vi "Measure Resistance (2 or 4-wire)_demo.vi"() -> ()   [LabVIEW 2013]
doc: "This example acquires a single Resistance measurement. Set the measurement type to either a 2-wire or 4-wire resistance measurement. Specify the range and absolute resolution of your input signal. The measured value will be displayed in the Measurement indicator. A Boolean indicator will indicate if the measured value is out of range."
uses:
  <instrlib>/niDMM/nidmm.llb/niDMM Function.ctl
  <instrlib>/niDMM/nidmm.llb/niDMM Resolution in Digits.ctl
  <instrlib>/niDMM/nidmm.llb/niDMM Offset Comp Ohms.ctl
  <instrlib>/niDMM/nidmm.llb/niDMM Configure Measurement Digits.vi
panel:
  out "Configuration:Range":dbl
  in  "Resolution in Digits":T1=5.5 items=["3 1/2"=3.5, "4 1/2"=4.5, "5 1/2"=5.5, "6 1/2"=6.5, "7 1/2"=7.5]
  out "Signal Out of Range":bool
  in  "Measurement Type":T2=enum."4-wire Resistance"
  in  "Device Name":refnum<k15>="4082_0"
  in  "Range (Ohms)":dbl=100.0 format="%.2p"
  out "Measurement (Ohms)":dbl format="%_7p"
  # "For instructions select File >> VI Properties >> Documentation"
  # "Configuration"
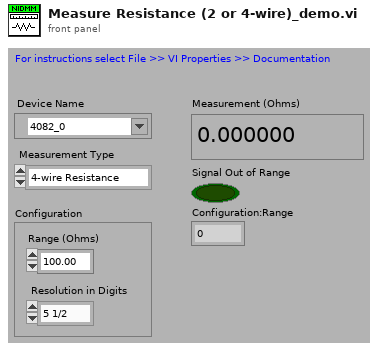
[diagram p1: front panel]
types:
  T1 = typedef "niDMM Resolution in Digits.ctl" = dbl
  T2 = typedef "niDMM Function.ctl" = enum16{"DC Volts", "AC Volts", "DC Current", "AC Current", "2-wire Resistance", "4-wire Resistance", "Diode", "Frequency", "Period", "AC Volts DC Coupled", "Capacitance", "Inductance", "Temperature"}
  T3 = typedef "niDMM Offset Comp Ohms.ctl" = i32
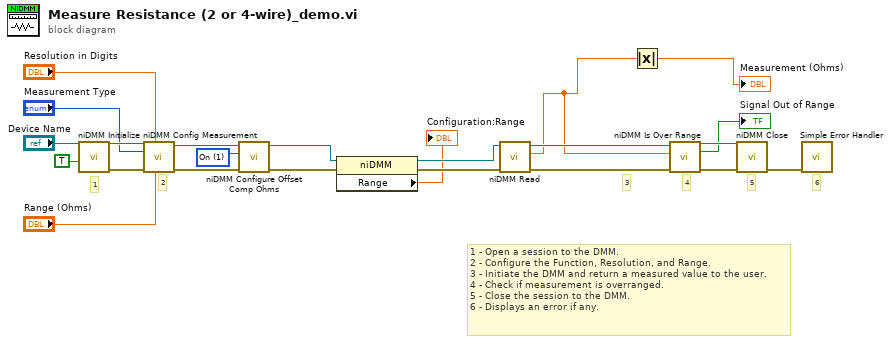
[diagram p0: block diagram]
diagram:
  w9 = T3 1 items=["Off", "On"] ("Offset Compensated Ohms")
  # "3"
  # "1 - Open a session to the DMM.\n2 - Configure the Function, Resolution, and Range.\n3 - Initiate the DMM and return a measured value to the user.\n4 - Check if measurement is overranged.\n5 - Close the session to the DMM.\n6 - Displays an error if any."
  # "1"
  # "6"
  # "5"
  # "4"
  # "2"
  n1 = call <instrlib>:"niDMM Initialize.vi"("Reset"=TRUE, "Instrument Descriptor"="Device Name") -> ("error out"=w22:errorcluster, "instrument handle out"=w23:refnum<k15>)  [unwired: 8 in]
  n2 = call-poly <instrlib>:"niDMM Config Measurement.vi"("Range"="Range (Ohms)", "Resolution in Digits"="Resolution in Digits", "error in (no error)"=w22, "Function"="Measurement Type", "instrument handle"=w23) -> ("error out"=w11:errorcluster, "instrument handle out"=w10:refnum<k15>)  [unwired: 5 in]
  n3 = call <instrlib>:"niDMM Configure Offset Comp Ohms.vi"("error in (no error)"=w11, "Offset Compensated Ohms"=w9, "instrument handle"=w10) -> ("error out"=w5:errorcluster, "instrument handle out"=w4:refnum<k15>)  [unwired: 7 in]
  n4 = property class="niDMM"(reference=w4, error in=w5) -> (reference out=w2:refnum<k15>, error out=w3:errorcluster, "Range"=→"Configuration:Range":dbl)
  n5 = call <instrlib>:"niDMM Read.vi"("error in (no error)"=w3, "instrument handle"=w2) -> ("error out"=w13:errorcluster, "Measurement"=w8:dbl, "instrument handle out"=w12:refnum<k15>)  [unwired: 7 in]
  n6 = Absolute Value(x=w8) -> (abs(x)=→"Measurement (Ohms)":dbl)
  n7 = call <instrlib>:"niDMM Is Over Range.vi"("error in (no error)"=w13, "Measurement"=w8, "instrument handle"=w12) -> ("error out"=w17:errorcluster, "Over Range?"=→"Signal Out of Range":bool, "instrument handle out"=w18:refnum<k15>)  [unwired: 6 in]
  n8 = call <instrlib>:"niDMM Close.vi"("error in (no error)"=w17, "instrument handle"=w18) -> ("error out"=w16:errorcluster)  [unwired: 9 in]
  n9 = call <vilib>:"Simple Error Handler.vi"("error in (no error)"=w16) -> ()  [unwired: 4 in, 5 out]
